vi "Generate DC Voltage.vi"(9 "Lines in (String)":string="Dev1/ao2", 10 "Device Name":string, 11 "Voltage":dbl format="%0.2f") -> (0 "error out":errorcluster)   [LabVIEW 2013]
doc: "This example demonstrates how to generate a user-defined voltage using the analog output of a DAQ device."
uses:
  <vilib>/DAQmx/create/channels.llb/DAQmx Create Channel (AO-Voltage-Basic).vi
  <vilib>/DAQmx/write.llb/DAQmx Write (Analog DBL 1Chan 1Samp).vi
panel:
  in  "Max Voltage":dbl=10.0
  in  "Min Voltage":dbl
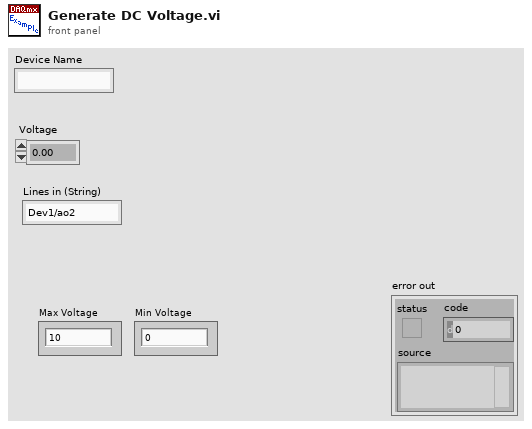
[diagram p1: front panel]
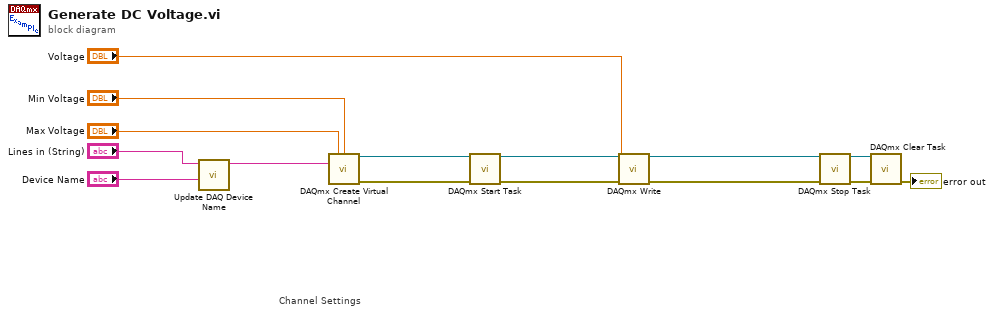
[diagram p0: block diagram]
diagram:
  # "Channel Settings"
  n1 = call "Update DAQ Device Name.vi"("Device Name"="Device Name", "Lines in (String)"="Lines in (String)") -> ("Lines out"=w4:tag)  [unwired: 9 in]
  n2 = call-poly <vilib>:"DAQmx Create Virtual Channel.vi"("maximum value"="Max Voltage", "minimum value"="Min Voltage", "physical channels"=w4) -> ("task out"=w13:refnum<k21>, "error out"=w12:errorcluster)  [unwired: 11 in]
  n3 = call <vilib>:"DAQmx Start Task.vi"("task/channels in"=w13, "error in"=w12) -> ("task out"=w11:refnum<k21>, "error out"=w10:errorcluster)  [unwired: 12 in]
  n4 = call-poly <vilib>:"DAQmx Write.vi"("task/channels in"=w11, "data"="Voltage", "error in"=w10) -> ("task out"=w9:refnum<k21>, "error out"=w8:errorcluster)  [unwired: 10 in, 1 out]
  n5 = call <vilib>:"DAQmx Stop Task.vi"("task/channels in"=w9, "error in"=w8) -> ("task out"=w7:refnum<k21>, "error out"=w6:errorcluster)  [unwired: 12 in]
  n6 = call <vilib>:"DAQmx Clear Task.vi"("task in"=w7, "error in"=w6) -> ("error out"=→"error out":errorcluster)  [unwired: 13 in]
